vi "transfer_curve_dimension_with_burnin.vi"(0 "File Path":path, 1 "V_G Start":dbl=-0.7 format="%#.3g", 2 "V_G Finish":dbl=0.4 format="%#.3g", 3 "V_G Step Size":dbl=0.05 format="%#.3g", 4 "Preread delay (ms)":dbl=10000.0 format="%.2f", 5 "Delay between \naverages (ms)":dbl=200.0 format="%#.3f", 6 "Keithley 237 GPIB address":string="17", 7 "Software Averages":i16=5, 8 "VISA resource name":refnum<visa-resource-name>="GPIB0::25::INSTR", 9 "First bias settle (ms)":dbl=60000.0 format="%#.2f", 11 "Current Compliance\nLimit (A) Ke2400":dbl=1.0 format="%#.3e", 12 "Dimension(No.:1-8)":fxp<+,8,8>=1.0 caption="Dimension", 17 "Voltage Compliance Limit 237 (V)":dbl=10.0 format="%#.3f", 18 "Current Compliance\nLimit 237 (A)":dbl=0.1 format="%#.3f", 19 "V_DS":dbl=-0.6 format="%#_13g") -> ()   [LabVIEW 2018]
uses:
  <vilib>/Utility/file.llb/Write Delimited Spreadsheet (string).vi
  Instance           1 16Saved   JV curve .vi
  Program Files/National Instruments/LabVIEW 2017/instr.lib/ke237/KE237.LLB/Keith 237 Operate/Standby.vi
  <instrlib>/Keithley 24XX/Public/Data/Read (Single Point).vi
  <vilib>/Analysis/NI_AALBase.lvlib
  <instrlib>/Keithley 24XX/Keithley 24XX.lvlib
panel:
  in  "Quick Burn In?":bool
  out "timer":dbl format="%#_6f"
  out "Keithley 2400":cluster{dbl[], dbl[]}(graph)={[-2.0, -1.9, -1.8, -1.7, -1.6, -1.5], [-6.6965744e-11, -6.7804984e-11, -6.685451799999999e-11, -6.6450076e-11, -6.5125542e-11, -6.7339852e-11]}
  out "I_G (A)":dbl=-6.642986e-11 format="%.2e"
  in  "Autozero?":u16(ring) items=["On", "Off", "Once"]
  in  "Measurement Speed (1 PLC)":dbl=1.0 format="%.2g"
  in  "Manual Range (Max I)":dbl=1.0
  in  "Enable Meas Auto Range":bool=TRUE
  in  "Source Mode":u16(ring) items=["Voltage", "Current"]
  in  "Return Sweep?":bool=TRUE
  out "I_DS":dbl=-1.38e-12 format="%.2e"
  out "Outputfile":path=path "C:/DATA/Mark Ziffer/test10"
  in  "Abort Scan":bool=TRUE
  out "V_G":dbl=-1.5 format="%#.2f"
  out "Keithley 237":cluster{dbl[], dbl[]}(graph)={[-2.0, -1.9, -1.8, -1.7, -1.6, -1.5], [-6.720000000000001e-13, -2.18e-13, -2.7599999999999993e-13, -8.999999999999998e-14, -1.3999999999999998e-13, -1.3800000000000002e-13]}
  # "Transfer Curve\nbased on  EL_photocurrent_JV.vi for controlling 2 Ketthleys\n\n9/2017 MZ"
  # "Software Settings"
  # "Ke237 Settings"
  # "Ke2400 Settings"
  # "Notes for IV Scan\n\n2010.07.06 - add absolute value plotter to look at log-scale current\n2010.01.07 - Modified file headers for distinguihing when imported to Igor Pro - the prefix of each header will be the file name.\n2009.01.15 - I updated the code to run on the VISA driver convention. I also modified the file saving and the option to set the\n                      graph display.\n2008.12.01 - I fixed an issue with calculations of J. It was mis-wired to divide current by wavelength, rather than active area.  BM\n\n=========================\nI added the functionality to calculate the fill factor, rectification ratio, short circuit current density, and open circuit voltage. \nAdditionally, current density (mA/cm^2) is reported in the plot window and column B of the data file, and the current (A) has been \nmoved to column C. Open circuit voltage is linearly interpolated. The max power point (mpp) for calculating fill factor is taken as \nthe data point with the highest I-V product, so this makes it only as accurate as your voltage step size, but should be fine for a decent \ndevice on the 50 mV default step size.\n\nIf you know how to use the previous versions of IV scan, \nmake sure you set these parameters before you scan:\n1) Recftification Ratio Bias - this is the +/- bias value you wish to record a rectification ratio at.\n2) Effective Area - this is the area in cm^2 of the diode mask (photoactive area) when measuring under illumination or the measured \n     area of the electrode overlap when measured in dark (regular active area).\n3) Do you want to record a separate data file for the calculated characteristics? If so, make sure the switch is on.\n\nAs of today, I couldn't figure out how to append the computed characteristics to the I-V file without experiencing formating issues, so\nI opted to just create a separate file if you want to save that info. Feel free to fix this if you know how. Check tab 3 > tab 2 > tab 9 in the\nblock diagram.\n\n2008-04-15\nB MacLeod"
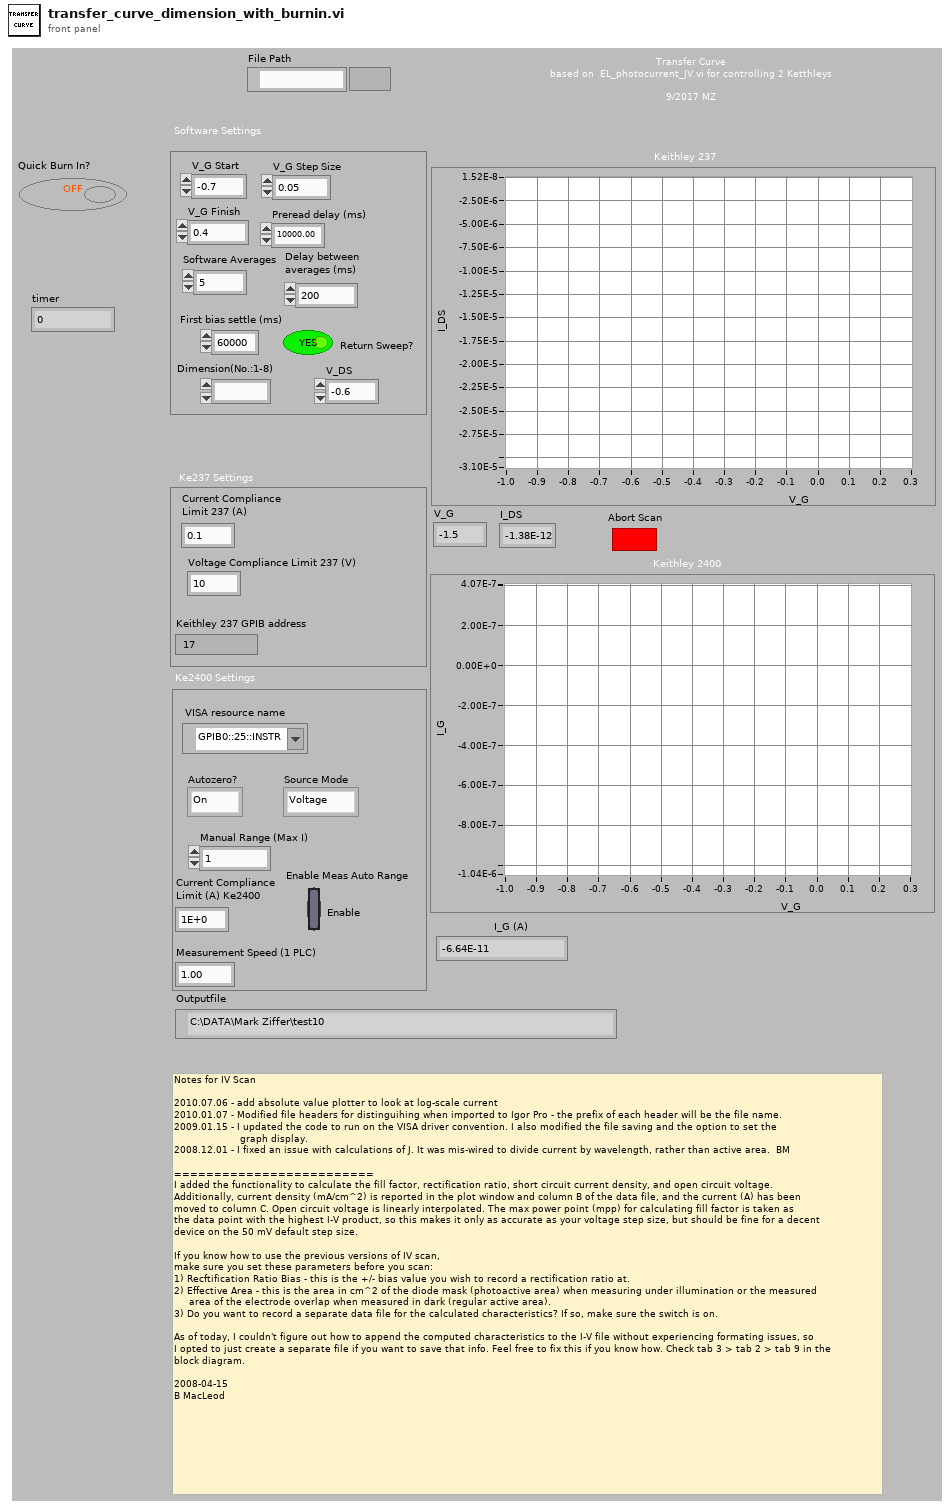
[diagram p1: front panel]
types:
  T1 = cluster{"error":bool, "code":i32, "source":string}
  T2 = cluster{"source value":string, "measure value":string, "delay value (sec)":string, "time value (sec)":string}[]
  T3 = cluster{"source value":dbl, "measure value":dbl, "delay value (sec)":dbl, "time value (sec)":dbl}[]
  T4 = cluster{"[0]":cluster{"source value":dbl, "measure value":dbl, "delay value (sec)":dbl, "time value (sec)":dbl}, "[1]":cluster{"source value":dbl, "measure value":dbl, "delay value (sec)":dbl, "time value (sec)":dbl}, "[2]":cluster{"source value":dbl, "measure value":dbl, "delay value (sec)":dbl, "time value (sec)":dbl}, "[3]":cluster{"source value":dbl, "measure value":dbl, "delay value (sec)":dbl, "time value (sec)":dbl}, "[4]":cluster{"source value":dbl, "measure value":dbl, "delay value (sec)":dbl, "time value (sec)":dbl}, "[5]":cluster{"source value":dbl, "measure value":dbl, "delay value (sec)":dbl, "time value (sec)":dbl}, "[6]":cluster{"source value":dbl, "measure value":dbl, "delay value (sec)":dbl, "time value (sec)":dbl}, "[7]":cluster{"source value":dbl, "measure value":dbl, "delay value (sec)":dbl, "time value (sec)":dbl}, "[8]":cluster{"source value":dbl, "measure value":dbl, "delay value (sec)":dbl, "time value (sec)":dbl}}
  T5 = cluster{"source value":dbl, "measure value":dbl, "delay value (sec)":dbl, "time value (sec)":dbl}
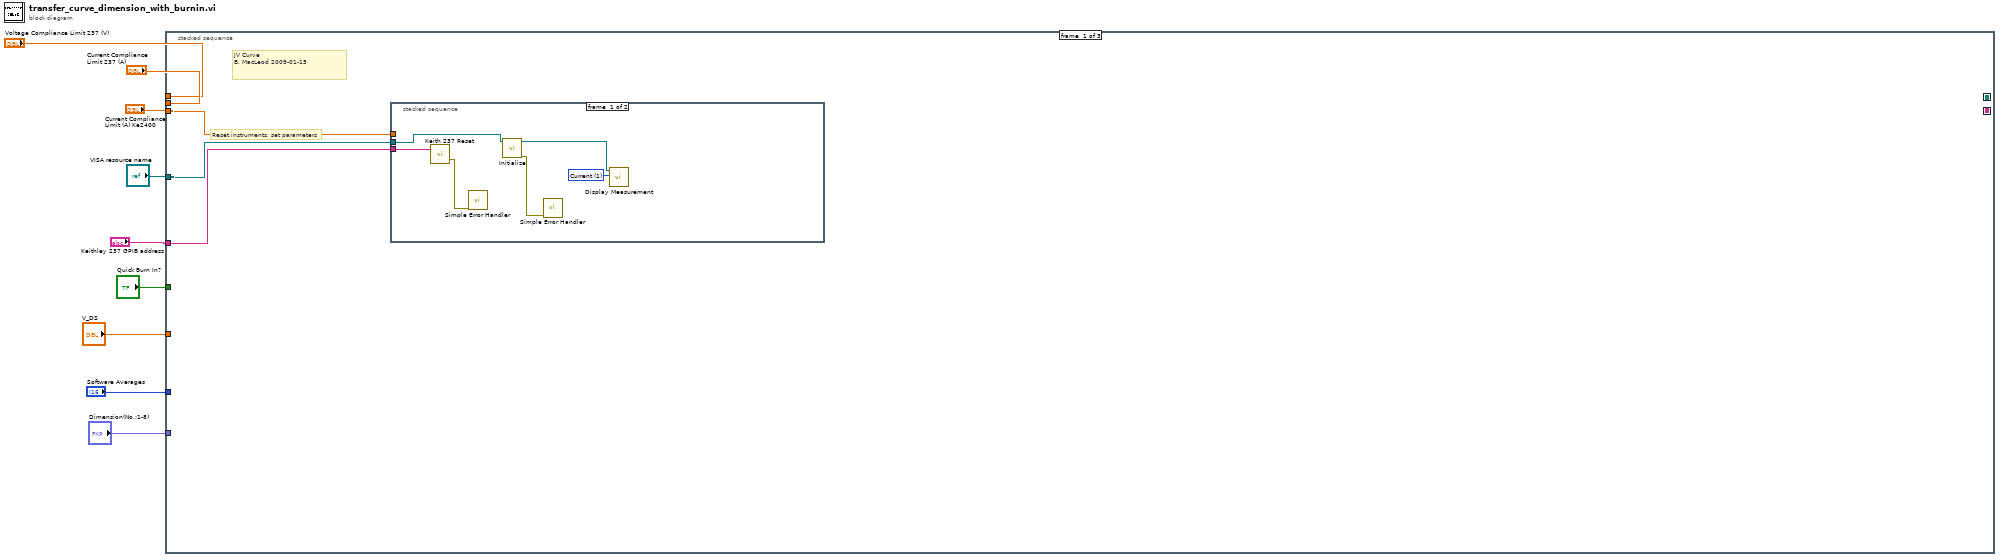
[diagram p0: block diagram]
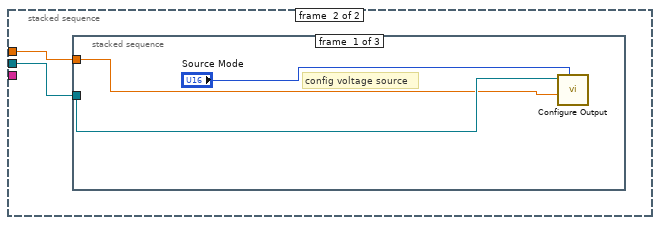
[diagram p2: hidden frame]
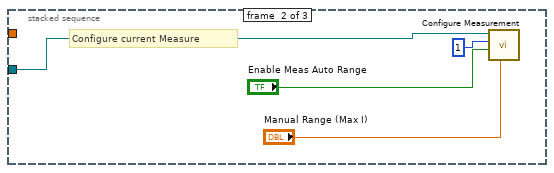
[diagram p3: hidden frame]
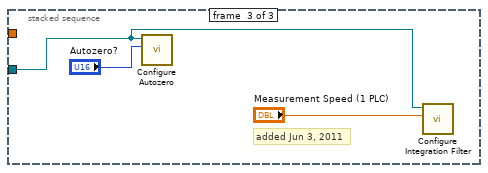
[diagram p4: hidden frame]
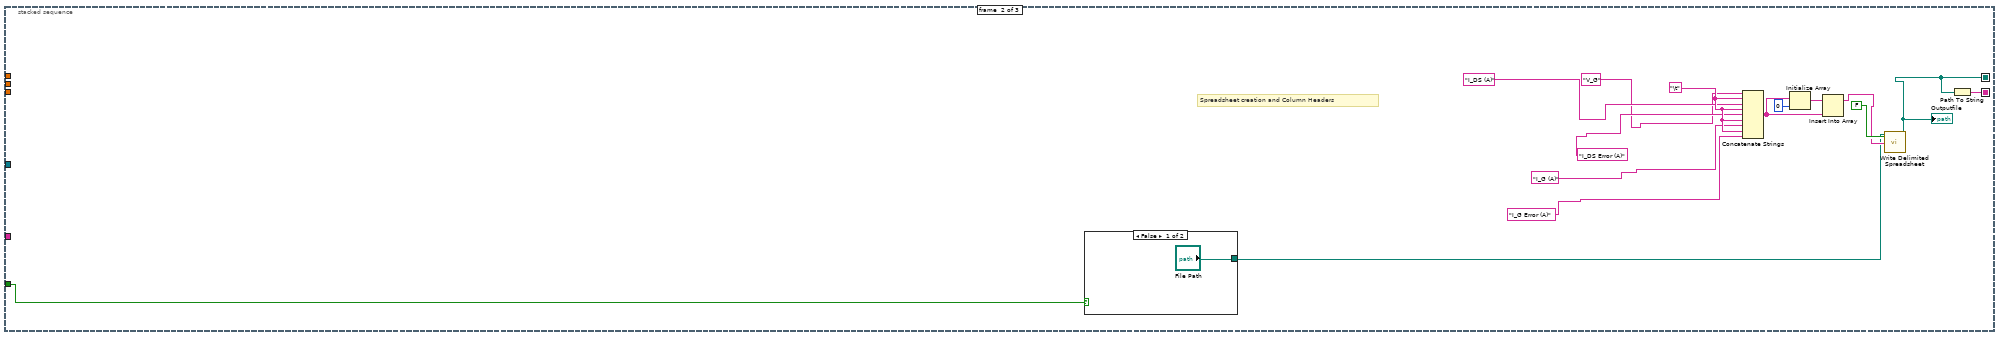
[diagram p5: hidden frame]
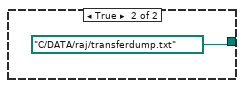
[diagram p6: hidden frame]
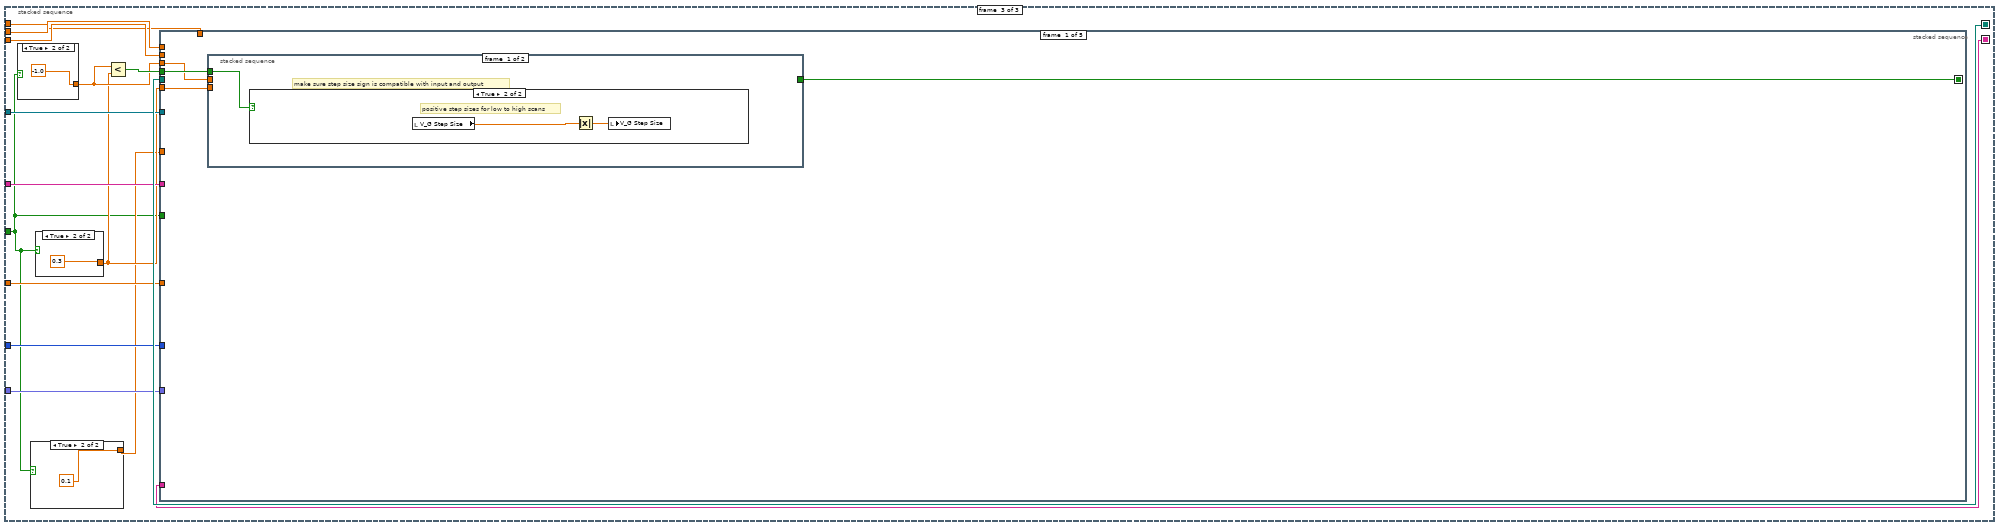
[diagram p7: hidden frame]
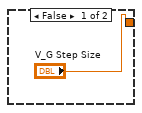
[diagram p8: hidden frame]
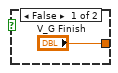
[diagram p9: hidden frame]
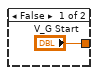
[diagram p10: hidden frame]
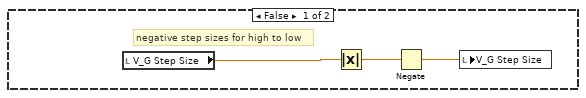
[diagram p11: hidden frame]
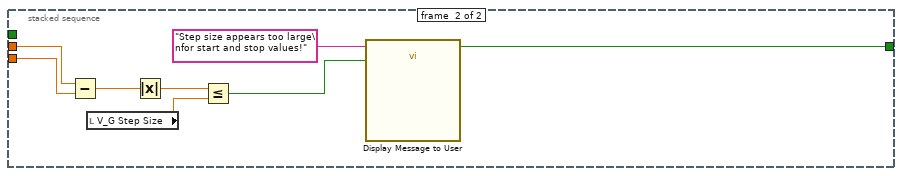
[diagram p12: hidden frame]
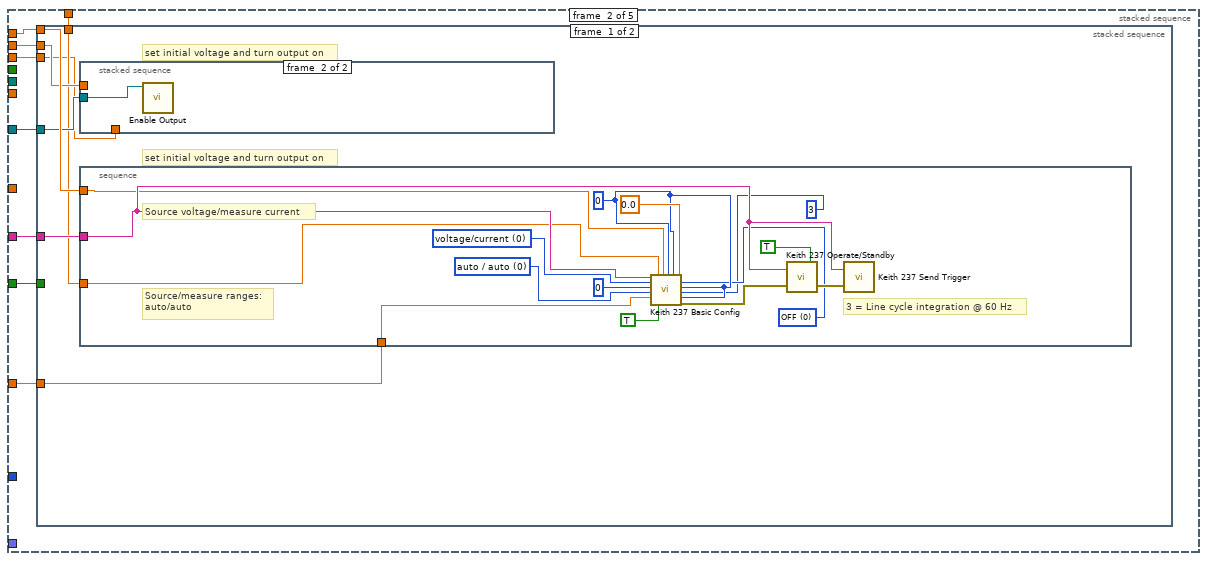
[diagram p13: hidden frame]
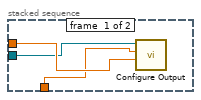
[diagram p14: hidden frame]
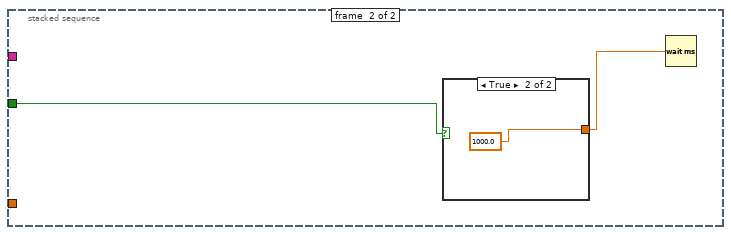
[diagram p15: hidden frame]
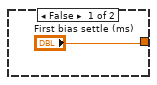
[diagram p16: hidden frame]
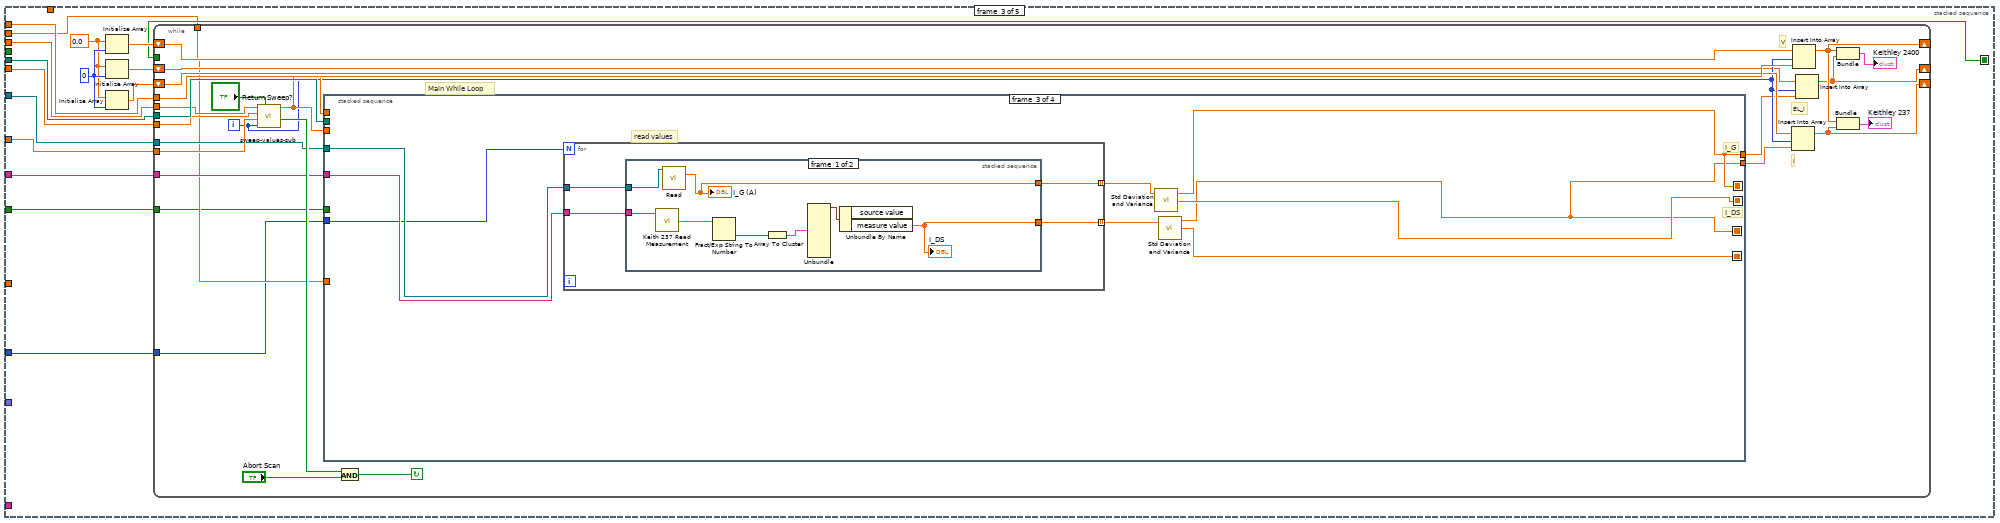
[diagram p17: hidden frame]
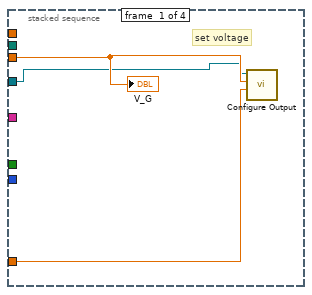
[diagram p18: hidden frame]
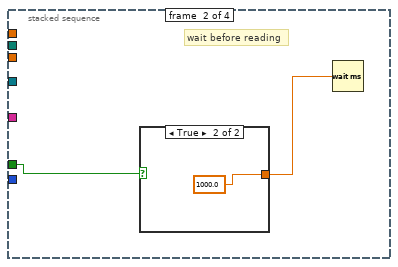
[diagram p19: hidden frame]
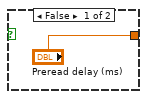
[diagram p20: hidden frame]
diagram:
  # "JV Curve\nB. MacLeod 2009-01-15"
  n1 = stacked-sequence {
    seq-local: [_ w38 _] -> [_ _ w61]
    seq-local: [_ w45 _] -> [_ _ w60]
    tunnel: "Current Compliance\nLimit 237 (A)" -> [_ _ w59]
    tunnel: "Voltage Compliance Limit 237 (V)" -> [_ _ w55]
    tunnel: "Keithley 237 GPIB address" -> [w12 _ w58]
    tunnel: "VISA resource name" -> [w11 _ w57]
    tunnel: "Current Compliance\nLimit (A) Ke2400" -> [w10 _ w56]
    tunnel: "V_DS" -> [_ _ w54]
    tunnel: "Software Averages" -> [_ _ w53]
    tunnel: "Dimension(No.:1-8)" -> [_ _ w52]
    tunnel: "Quick Burn In?" -> [_ w31 w48]
    frame #0 {
      # "Reset instruments, set parameters"
      n2 = stacked-sequence {
        tunnel: w12 -> [w17 _]
        tunnel: w11 -> [w16 w20]
        tunnel: w10 -> [_ w19]
        frame #0 {
          w15 = u16 1 items=["Voltage", "Current", "Resistance"] ("Displayed Measurement (0: Voltage)")
          n3 = call "Keith 237 Reset.vi"("GPIB address"=w17) -> ("error out"=w18:T1)  [unwired: 1 in]
          n4 = call <vilib>:"Simple Error Handler.vi"("error in (no error)"=w18) -> ()  [unwired: 1 in, 8 out]
          n5 = call <instrlib>:"Initialize.vi"("VISA resource name"=w16) -> ("error out"=w13:errorcluster, "VISA resource name out"=w14:refnum<visa-resource-name>)  [unwired: 9 in]
          n6 = call <vilib>:"Simple Error Handler.vi"("error in (no error)"=w13) -> ()  [unwired: 1 in, 8 out]
          n7 = call <instrlib>:"Display Measurement.vi"("Displayed Measurement (0: Voltage)"=w15, "VISA resource name"=w14) -> ()  [unwired: 8 in, 2 out]
        }
        frame #1 {
          n8 = stacked-sequence {
            tunnel: w20 -> [w22 w24 w28]
            tunnel: w19 -> [w21 _ _]
            frame #0 {
              # "config voltage source"
              n9 = call "Configure Output.vi"("Source Mode  (0: Voltage)"="Source Mode", "Compliance  Level (0.1)"=w21, "VISA resource name"=w22) -> ()  [unwired: 3 in, 6 out]
            }
            frame #1 {
              # "Configure current Measure"
              n10 = call "Configure Measurement.vi"("Manual Range (1.0)"="Manual Range (Max I)", "Enable Auto Range (T:Enable)"="Enable Meas Auto Range", "Function (0: Volts)"=1, "VISA resource name"=w24) -> ()  [unwired: 1 in, 7 out]
            }
            frame #2 {
              # "added Jun 3, 2011"
              n11 = call "Configure Autozero.vi"("Autozero  (0: On)"="Autozero?", "VISA resource name"=w28) -> ()  [unwired: 1 in, 9 out]
              n12 = call "Configure Integration Filter.vi"("Measurement Speed (1 PLC)"="Measurement Speed (1 PLC)", "VISA resource name"=w28) -> ()  [unwired: 8 in, 2 out]
            }
          }
        }
      }
    }
    frame #1 {
      w41 = "\t"
      # "Spreadsheet creation and Column Headers"
      n13 = case shown="False" w31 {
        tunnel: ["File Path" path "C:/DATA/raj/transferdump.txt"] -> w32
        frame False {
        }
        frame True {
        }
      }
      n14 = Concatenate Strings("V_G", w41, "I_DS (A)", w41, "I_DS Error (A)", w41, "I_G (A)", w41, "I_G Error (A)" ("string")) -> (w43:string)
      n15 = Initialize Array(w43, 0 ("dimension size")) -> (w42:string[])
      n16 = Insert Into Array(array=w42, new element=w43) -> (w39:string[])  [unwired: 1 in]
      n17 = call-poly <vilib>:"Write Delimited Spreadsheet.vi"("file path (dialog if empty)"=w32, "1D data"=w39, "transpose? (no:F)"=FALSE ("append to file? (new file:F)")) -> ("new file path (Not A Path if cancelled)"=w38:path)  [unwired: 11 in, 1 out]
      "Outputfile" <- w38
      n18 = Path To String(path=w38) -> (string=w45:string)
    }
    frame #2 {
      n19 = case shown="True" w48 {
        tunnel: ["V_G Start" -1.0] -> w51
        frame False {
        }
        frame True {
        }
      }
      n20 = case shown="True" w48 {
        tunnel: ["V_G Step Size" 0.1] -> w49
        frame False {
        }
        frame True {
        }
      }
      n21 = case shown="True" w48 {
        tunnel: ["V_G Finish" 0.3] -> w50
        frame False {
        }
        frame True {
        }
      }
      n22 = Less?(x=w51, y=w50) -> (x < y?=w62:bool)
      n23 = stacked-sequence {
        seq-local: [w69 _ _ _ _] -> [_ _ w133 _ _]
        tunnel: w62 -> [w72 _ _ _ _]
        tunnel: w51 -> [w71 w89 w139 _ _]
        tunnel: w50 -> [w70 _ w140 _ _]
        tunnel: w49 -> [_ _ w138 _ _]
        tunnel: w61 -> [_ _ w137 w217 _]
        tunnel: w60 -> [_ _ _ _ _]
        tunnel: w59 -> [_ w94 w134 _ _]
        tunnel: w58 -> [_ w93 w132 _ w275]
        tunnel: w57 -> [_ w91 w131 _ w274]
        tunnel: w56 -> [_ w92 w127 _ _]
        tunnel: w55 -> [_ w90 _ _ _]
        tunnel: w54 -> [_ w88 _ w218 _]
        tunnel: w53 -> [_ _ w126 w216 _]
        tunnel: w52 -> [_ _ _ w213 _]
        tunnel: w48 -> [_ w87 w125 _ _]
        frame #0 {
          n24 = stacked-sequence {
            tunnel: w72 -> [w73 _]
            tunnel: w71 -> [_ w86]
            tunnel: w70 -> [_ w85]
            tunnel: [_ w79] -> w69
            frame #0 {
              # "make sure step size sign is compatible with input and output"
              n25 = case shown="True" w73 {
                frame False {
                  # "negative step sizes for high to low"
                  n26 = local read "V_G Step Size"() -> (w76:dbl)
                  n27 = Absolute Value(x=w76) -> (abs(x)=w75:dbl)
                  n28 = Negate(x=w75) -> (-x=w74:dbl)
                  n29 = local write "V_G Step Size"(w74) -> ()
                }
                frame True {
                  # "positive step sizes for low to high scans"
                  n30 = local read "V_G Step Size"() -> (w78:dbl)
                  n31 = Absolute Value(x=w78) -> (abs(x)=w77:dbl)
                  n32 = local write "V_G Step Size"(w77) -> ()
                }
              }
            }
            frame #1 {
              n33 = Subtract(x=w86, y=w85) -> (x-y=w84:dbl)
              n34 = local read "V_G Step Size"() -> (w82:dbl)
              n35 = Absolute Value(x=w84) -> (abs(x)=w83:dbl)
              n36 = Less Or Equal?(x=w83, y=w82) -> (x <= y?=w80:bool)
              n37 = call "Display Message to User"("Enable"=w80, "Message"="Step size appears too large\nfor start and stop values!") -> ("OK"=w79:bool)  [unwired: 1 in, 8 out]
            }
          }
        }
        frame #1 {
          n38 = stacked-sequence {
            tunnel: w94 -> [w101 _]
            tunnel: w93 -> [w100 _]
            tunnel: w92 -> [w99 _]
            tunnel: w91 -> [w98 _]
            tunnel: w90 -> [w97 _]
            tunnel: w89 -> [w96 _]
            tunnel: w88 -> [w95 _]
            tunnel: w87 -> [_ w122]
            frame #0 {
              # "set initial voltage and turn output on"
              # "set initial voltage and turn output on"
              n39 = stacked-sequence {
                tunnel: w99 -> [w104 _]
                tunnel: w98 -> [w103 w105]
                tunnel: w96 -> [w102 _]
                frame #0 {
                  n40 = call "Configure Output.vi"("Compliance  Level (0.1)"=w104, "Output Level (0)"=w102, "VISA resource name"=w103) -> ()  [unwired: 3 in, 6 out]
                }
                frame #1 {
                  n41 = call "Enable Output.vi"("VISA resource name"=w105) -> ()  [unwired: 2 in, 9 out]
                }
              }
              n42 = stacked-sequence {
                tunnel: w101 -> [w109]
                tunnel: w100 -> [w111]
                tunnel: w97 -> [w108]
                tunnel: w95 -> [w106]
                frame #0 {
                  w110 = u16 0 items=["OFF", "ON"] ("default delay (on:1)")
                  w112 = u16 0 items=["auto / auto", "1 nA / 1.1 V", "10 nA / 11 V", "100 nA / 110 V", "0.001 mA / 1100 V", "0.01 mA / 1100 V", "0.1 mA / 1100 V", "1 mA / 1100 V", "10 mA / 1100 V", "100 mA / 1100 V"] ("source range\nI source / V source (auto:0)")
                  w113 = u16 0 items=["voltage/current", "current/voltage"] ("source/measure (V/I:0)")
                  w115 = u16 0
                  # "3 = Line cycle integration @ 60 Hz"
                  # "Source/measure ranges:\nauto/auto"
                  # "Source voltage/measure current"
                  n43 = call "Keith 237 Basic Config.vi"("GPIB address"=w111, "source/measure (V/I:0)"=w113, "function (DC:0)"=u16 0, "source range\nI source / V source (auto:0)"=w112, "source level"=w106, "voltage \ncompliance level"=w108, "1100 V range (disabled:F)"=TRUE, "current \ncompliance level"=w109, "compliance/\nmeasurement range (auto:0)"=w115, "suppression (off:0)"=w115, "DC delay (sec)"=0.0, "default delay (on:1)"=w110, "filter (disabled:0)"=w115, "integration time (medium:1)"=u16 3, "sense (local:0)"=w115) -> ("error out"=w120:T1)  [unwired: 4 in]
                  n44 = call "Keith 237 Operate/Standby.vi"("source"=TRUE, "error in"=w120, "GPIB address"=w111) -> ("error out"=w118:T1)
                  n45 = call "Keith 237 Send Trigger.vi"("GPIB address"=w111, "error in"=w118) -> ()  [unwired: 1 out]
                }
              }
            }
            frame #1 {
              n46 = case shown="True" w122 {
                tunnel: ["First bias settle (ms)" 1000.0] -> w121
                frame False {
                }
                frame True {
                }
              }
              n47 = Wait (ms)(milliseconds to wait=w121) -> ()  [unwired: 1 out]
            }
          }
        }
        frame #2 {
          w130 = 0
          w129 = 0.0
          n48 = Initialize Array(w129, w130) -> (w136:dbl[])
          n49 = Initialize Array(w129, w130) -> (w128:dbl[])
          n50 = Initialize Array(w129, w130) -> (w135:dbl[])
          n51 = while {
            shift-left: w135 -> [w162]
            shift-right: [w150] -> _
            shift-left: w136 -> [w163]
            shift-right: [w153] -> _
            tunnel: w137 -> [w165]
            tunnel: w138 -> [w161]
            tunnel: w139 -> [w160]
            tunnel: w140 -> [w159]
            tunnel: w134 -> [w157]
            tunnel: w133 -> [_]
            shift-right: [w149] -> _
            shift-left: w128 -> [w145]
            tunnel: w132 -> [w148]
            tunnel: w131 -> [w147]
            tunnel: w127 -> [w143]
            tunnel: w126 -> [w142]
            tunnel: w125 -> [w141]
            i -> [w151]
            stop <- w155 continue-if-true
            # "EL_I"
            # "Main While Loop"
            # "V"
            # "I"
            n52 = call "sweep-values-sub.vi"("Forward/Reverse"="Return Sweep?", "Point Number"=w151, "Step Size"=w161, "Sweep Stop"=w159, "Sweep Start"=w160) -> ("Active"=w156:bool, "Output"=w164:dbl)  [unwired: 2 out]
            n53 = stacked-sequence {
              seq-local: [_ _ w182 _] -> [_ _ _ w199]
              seq-local: [_ _ w176 _] -> [_ _ _ w200]
              seq-local: [_ _ w178 _] -> [_ _ _ w198]
              seq-local: [_ _ w177 _] -> [_ _ _ w197]
              tunnel: [_ _ w176 _] -> w152
              tunnel: w164 -> [w169 _ _ w211]
              tunnel: w165 -> [_ _ _ w202]
              tunnel: w157 -> [_ _ _ _]
              tunnel: w148 -> [_ _ w180 _]
              tunnel: w147 -> [w167 _ w179 _]
              tunnel: [_ _ w178 _] -> w146
              tunnel: w143 -> [w168 _ _ _]
              tunnel: w142 -> [_ _ w175 _]
              tunnel: w141 -> [_ w170 _ _]
              frame #0 {
                # "set voltage"
                n54 = call "Configure Output.vi"("Compliance  Level (0.1)"=w168, "Output Level (0)"=w169, "VISA resource name"=w167) -> ()  [unwired: 3 in, 6 out]
                "V_G" <- w169
              }
              frame #1 {
                # "wait before reading"
                n55 = case shown="True" w170 {
                  tunnel: ["Preread delay (ms)" 1000.0] -> w171
                  frame False {
                  }
                  frame True {
                  }
                }
                n56 = Wait (ms)(milliseconds to wait=w171) -> ()  [unwired: 1 out]
              }
              frame #2 {
                # "I_DS"
                # "I_G"
                # "read values"
                n57 = for {
                  N: w175 -> [_]
                  tunnel: [w186] -> w181 mode=indexing
                  tunnel: w180 -> [w185]
                  tunnel: w179 -> [w184]
                  tunnel: [w183] -> w174 mode=indexing
                  n58 = stacked-sequence {
                    tunnel: [w191 _] -> w186
                    tunnel: w185 -> [w189 _]
                    tunnel: w184 -> [w188 _]
                    tunnel: [w187 _] -> w183
                    frame #0 {
                      n59 = call "Keith 237 Read Measurement.vi"("GPIB address"=w189) -> ("display"=w194:T2)  [unwired: 1 in, 3 out]
                      n60 = call-poly <instrlib>:"Read.vi"("VISA resource name"=w188) -> ("Current"=w187:sgl)  [unwired: 8 in, 6 out]
                      "I_G (A)" <- w187
                      n61 = Fract/Exp String To Number(string=w194) -> (number=w190:T3)  [unwired: 3 in, 1 out]
                      n62 = Array To Cluster(array=w190) -> (cluster=w193:T4)
                      n63 = Unbundle(w193) -> ("[0]"=w192:T5)  [unwired: 8 out]
                      n64 = Unbundle By Name(w192) -> ("measure value"=w191:dbl)  [unwired: 1 out]
                      "I_DS" <- w191
                    }
                    frame #1 {
                      n65 = Wait (ms)(milliseconds to wait="Delay between \naverages (ms)") -> (millisecond timer value=→"timer":u32)
                    }
                  }
                }
                n66 = call <vilib>:"Std Deviation and Variance.vi"("X"=w174) -> ("mean"=w178:dbl, "standard deviation"=w177:dbl)  [unwired: 1 in, 1 out]
                n67 = call <vilib>:"Std Deviation and Variance.vi"("X"=w181) -> ("mean"=w176:dbl, "standard deviation"=w182:dbl)  [unwired: 1 in, 1 out]
              }
              frame #3 {
                w206 = "\t"
                # "I_G"
                # "write data to file"
                # "X"
                n68 = Format Into String(format string="%#f", w211) -> (resulting string=w209:string)  [unwired: 2 in, 1 out]
                n69 = Number To Exponential String(number=w200) -> (E-format string=w212:string)  [unwired: 3 out]
                n70 = Number To Exponential String(number=w199) -> (E-format string=w208:string)  [unwired: 3 out]
                n71 = Number To Exponential String(number=w198) -> (E-format string=w205:string)  [unwired: 3 out]
                n72 = Number To Exponential String(number=w197) -> (E-format string=w204:string)  [unwired: 3 out]
                n73 = Concatenate Strings(w209, w206, w212, w206, w208, w206, w205, w206, w204) -> (w207:string)
                n74 = Build Array(w207) -> (w203:string[])
                n75 = call-poly <vilib>:"Write Delimited Spreadsheet.vi"("file path (dialog if empty)"=w202, "1D data"=w203, "append to file? (new file:F)"=TRUE) -> ()  [unwired: 11 in, 2 out]
              }
            }
            n76 = Compound Arithmetic op=AND(w156, "Abort Scan") -> (w155:bool)
            n77 = Insert Into Array(array=w162, index=w151, new element=w152) -> (w150:dbl[])
            n78 = Insert Into Array(array=w163, index=w151, new element=w164) -> (w153:dbl[])
            n79 = Insert Into Array(array=w145, index=w151, new element=w146) -> (w149:dbl[])
            n80 = Bundle(w153, w149) -> (→"Keithley 2400":cluster{dbl[], dbl[]})  [unwired: 1 out]
            n81 = Bundle(w153, w150) -> (→"Keithley 237":cluster{dbl[], dbl[]})  [unwired: 1 out]
          }
        }
        frame #3 {
          n82 = case shown="5" w213 {
            tunnel: [100 100 100 100 2000 1000 200 50] -> w215
            tunnel: [20 20 20 20 20 20 20 20] -> w214
            frame 1, Default {
            }
            frame 2 {
            }
            frame 3 {
            }
            frame 4 {
            }
            frame 5 {
            }
            frame 6 {
            }
            frame 7 {
            }
            frame 8 {
            }
          }
          n83 = stacked-sequence {
            tunnel: w218 -> [_ w246 _ _ _]
            tunnel: w217 -> [w235 w244 w250 w265 w267]
            tunnel: w216 -> [_ _ w252 _ _]
            tunnel: w215 -> [_ _ _ w260 _]
            tunnel: w214 -> [_ _ _ _ w266]
            frame #0 {
              w240 = ""
              w239 = "\t"
              n84 = Concatenate Strings(w240, w239, w240, w239) -> (w236:string)
              n85 = Build Array(w236) -> (w238:string[])
              n86 = call-poly <vilib>:"Write Delimited Spreadsheet.vi"("file path (dialog if empty)"=w235, "1D data"=w238, "append to file? (new file:F)"=TRUE) -> ()  [unwired: 11 in, 2 out]
            }
            frame #1 {
              w247 = "\t"
              n87 = Number To Fractional String(number=w246, precision (6)=3) -> (F-format string=w245:string)  [unwired: 2 in]
              n88 = Concatenate Strings("V_DS = ", w247, w245, w247) -> (w248:string)
              n89 = Build Array(w248) -> (w243:string[])
              n90 = call-poly <vilib>:"Write Delimited Spreadsheet.vi"("file path (dialog if empty)"=w244, "1D data"=w243, "append to file? (new file:F)"=TRUE) -> ()  [unwired: 11 in, 2 out]
            }
            frame #2 {
              w255 = "\t"
              n91 = Number To Decimal String(number=w252) -> (decimal integer string=w251:string)  [unwired: 1 in]
              n92 = Concatenate Strings("Number of Averages = ", w255, w251, w255) -> (w256:string)
              n93 = Build Array(w256) -> (w254:string[])
              n94 = call-poly <vilib>:"Write Delimited Spreadsheet.vi"("file path (dialog if empty)"=w250, "1D data"=w254, "append to file? (new file:F)"=TRUE) -> ()  [unwired: 11 in, 2 out]
            }
            frame #3 {
              w262 = "\t"
              n95 = Number To Decimal String(number=w260) -> (decimal integer string=w261:string)  [unwired: 1 in]
              n96 = Concatenate Strings("Width/um =", w262, w261, w262) -> (w259:string)
              n97 = Build Array(w259) -> (w258:string[])
              n98 = call-poly <vilib>:"Write Delimited Spreadsheet.vi"("file path (dialog if empty)"=w265, "1D data"=w258, "append to file? (new file:F)"=TRUE) -> ()  [unwired: 11 in, 2 out]
            }
            frame #4 {
              w268 = "\t"
              n99 = Number To Decimal String(number=w266) -> (decimal integer string=w271:string)  [unwired: 1 in]
              n100 = Concatenate Strings("Length/um =", w268, w271, w268) -> (w272:string)
              n101 = Build Array(w272) -> (w273:string[])
              n102 = call-poly <vilib>:"Write Delimited Spreadsheet.vi"("file path (dialog if empty)"=w267, "1D data"=w273, "append to file? (new file:F)"=TRUE) -> ()  [unwired: 11 in, 2 out]
            }
          }
        }
        frame #4 {
          # "reset instrument at end of sweep"
          n103 = call <instrlib>:"Reset.vi"("VISA resource name"=w274) -> ()  [unwired: 9 in, 2 out]
          n104 = call "Keith 237 Reset.vi"("GPIB address"=w275) -> ()  [unwired: 1 in, 1 out]
        }
      }
    }
  }
